vi "String.CSV Spreadsheet String to 2D Array.vi"(1 "CSV Data":string) -> (0 "2D Data":string[][](array[string]))   [LabVIEW 2018]
uses:
  <vilib>/KATE/Strings/String Utils.lvlib
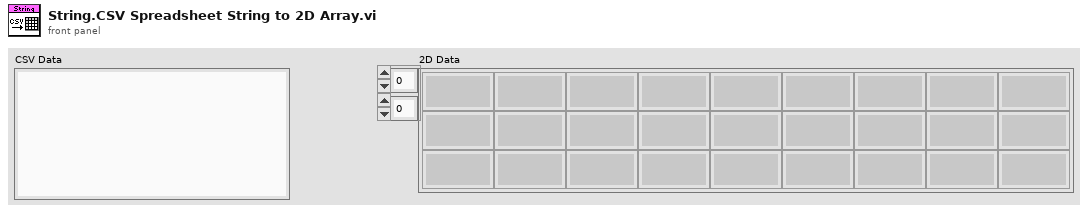
[diagram p1: front panel]
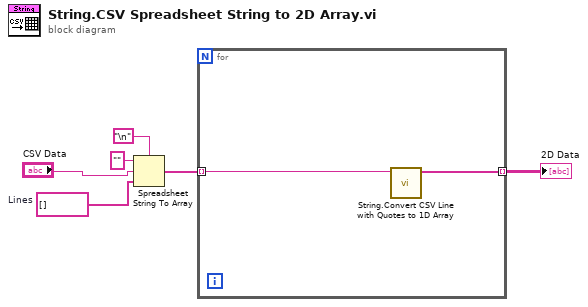
[diagram p0: block diagram]
diagram:
  w3 = string[] []  # Lines
  n1 = Spreadsheet String To Array(delimiter (Tab)="\n", format string="", spreadsheet string="CSV Data", array type (2D Dbl)=w3) -> (array=w2:string[])
  n2 = for {
    tunnel: w2 -> [w8] mode=indexing
    tunnel: [w7] -> w1 mode=indexing
    n3 = call <vilib>:"String.Convert CSV Line with Quotes to 1D Array.vi"("CSV String"=w8) -> ("Array"=w7:string[])  [unwired: 9 in, 1 out]
  }
  "2D Data" <- w1
